vi "set_LCD_init.vi"   [LabVIEW 2015]
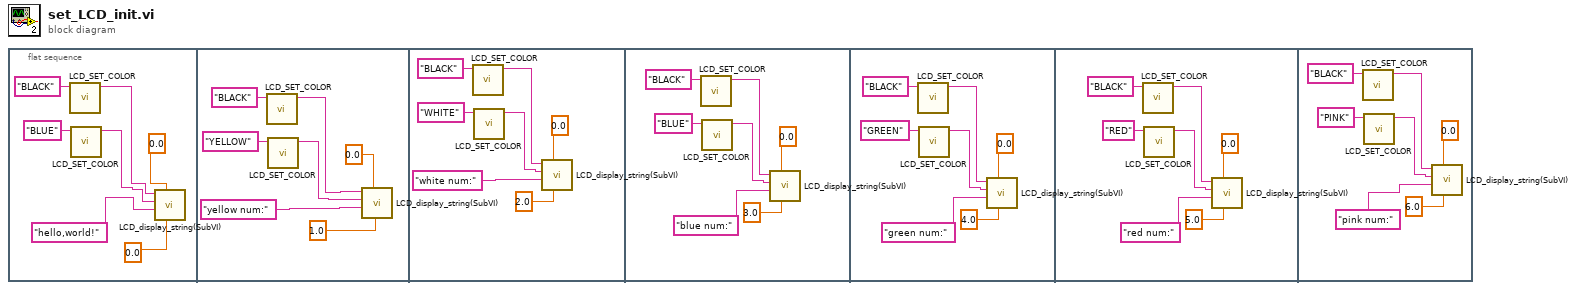
[diagram p0: block diagram]
diagram:
  n1 = flat-sequence {
    frame #0 {
      n2 = call "LCD_SET_COLOR.vi"("String in"="BLACK") -> ("String out"=w4:string)  [unwired: 10 in]
      n3 = call "LCD_SET_COLOR.vi"("String in"="BLUE") -> ("String out"=w3:string)  [unwired: 10 in]
      n4 = call "LCD_display_string(SubVI).vi"("y"=0.0, "x"=0.0, "String"="hello,world!", "char_color"=w3, "background"=w4) -> ()  [unwired: 7 in]
    }
    frame #1 {
      n5 = call "LCD_SET_COLOR.vi"("String in"="BLACK") -> ("String out"=w11:string)  [unwired: 10 in]
      n6 = call "LCD_SET_COLOR.vi"("String in"="YELLOW") -> ("String out"=w10:string)  [unwired: 10 in]
      n7 = call "LCD_display_string(SubVI).vi"("y"=1.0, "x"=0.0, "String"="yellow num:", "char_color"=w10, "background"=w11) -> ()  [unwired: 7 in]
    }
    frame #2 {
      n8 = call "LCD_SET_COLOR.vi"("String in"="BLACK") -> ("String out"=w19:string)  [unwired: 10 in]
      n9 = call "LCD_SET_COLOR.vi"("String in"="WHITE") -> ("String out"=w20:string)  [unwired: 10 in]
      n10 = call "LCD_display_string(SubVI).vi"("y"=2.0, "x"=0.0, "String"="white num:", "char_color"=w20, "background"=w19) -> ()  [unwired: 7 in]
    }
    frame #3 {
      n11 = call "LCD_SET_COLOR.vi"("String in"="BLACK") -> ("String out"=w24:string)  [unwired: 10 in]
      n12 = call "LCD_SET_COLOR.vi"("String in"="BLUE") -> ("String out"=w23:string)  [unwired: 10 in]
      n13 = call "LCD_display_string(SubVI).vi"("y"=3.0, "x"=0.0, "String"="blue num:", "char_color"=w23, "background"=w24) -> ()  [unwired: 7 in]
    }
    frame #4 {
      n14 = call "LCD_SET_COLOR.vi"("String in"="BLACK") -> ("String out"=w31:string)  [unwired: 10 in]
      n15 = call "LCD_SET_COLOR.vi"("String in"="GREEN") -> ("String out"=w30:string)  [unwired: 10 in]
      n16 = call "LCD_display_string(SubVI).vi"("y"=4.0, "x"=0.0, "String"="green num:", "char_color"=w30, "background"=w31) -> ()  [unwired: 7 in]
    }
    frame #5 {
      n17 = call "LCD_SET_COLOR.vi"("String in"="BLACK") -> ("String out"=w38:string)  [unwired: 10 in]
      n18 = call "LCD_SET_COLOR.vi"("String in"="RED") -> ("String out"=w37:string)  [unwired: 10 in]
      n19 = call "LCD_display_string(SubVI).vi"("y"=5.0, "x"=0.0, "String"="red num:", "char_color"=w37, "background"=w38) -> ()  [unwired: 7 in]
    }
    frame #6 {
      n20 = call "LCD_SET_COLOR.vi"("String in"="BLACK") -> ("String out"=w45:string)  [unwired: 10 in]
      n21 = call "LCD_SET_COLOR.vi"("String in"="PINK") -> ("String out"=w44:string)  [unwired: 10 in]
      n22 = call "LCD_display_string(SubVI).vi"("y"=6.0, "x"=0.0, "String"="pink num:", "char_color"=w44, "background"=w45) -> ()  [unwired: 7 in]
    }
  }
